vi "RPC Driver Library Path.vi"(8 "Driver ID (\"\")":string, 9 "Driver Type (\"\")":string, 10 "Base Path (empty)":path, 11 "App Ref (null: local)":refnum<vi>) -> (0 "Driver Config Name":string, 1 "Driver Component Name":string, 2 "Driver Library Path":path, 3 "dup App Ref":refnum<vi>)   [LabVIEW 2011]
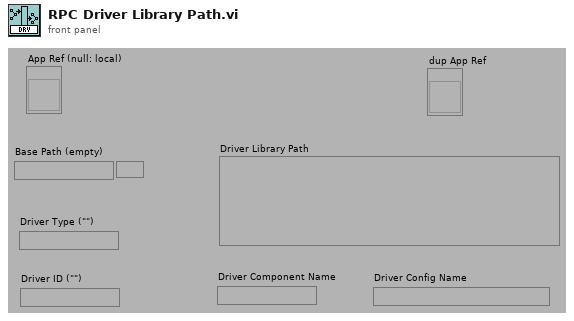
[diagram p1: front panel]
types:
  T1 = enum32{"invalid app kind", "Development System", "Run Time System", "Student Edition", "Embedded LabVIEW", "Evaluation", "Custom"}
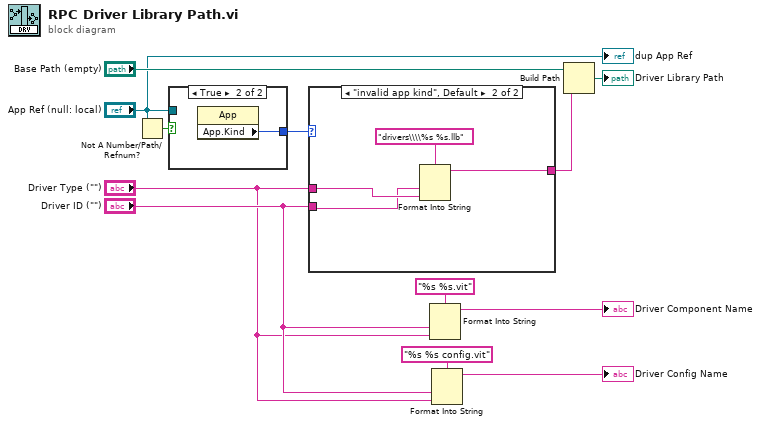
[diagram p0: block diagram]
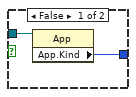
[diagram p2: hidden frame]
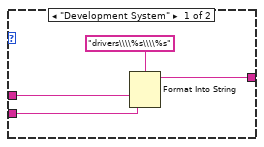
[diagram p3: hidden frame]
diagram:
  n1 = Not A Number/Path/Refnum?(number/path/refnum="App Ref (null: local)") -> (NaN/Path/Refnum?=w1:bool)
  n2 = case shown="True" w1 {
    tunnel: [w14 w15] -> w10
    tunnel: "App Ref (null: local)" -> [w13 _]
    frame False {
      n3 = property class="App"(reference=w13) -> ("App.Kind"=w14:T1)  [unwired: 1 in, 2 out]
    }
    frame True {
      n4 = property class="App"() -> ("App.Kind"=w15:T1)  [unwired: 2 in, 2 out]
    }
  }
  n5 = case shown="\"invalid app kind\", Default" w10 {
    tunnel: [w18 w22] -> w12
    tunnel: "Driver ID (\"\")" -> [w17 w20]
    tunnel: "Driver Type (\"\")" -> [w16 w21]
    frame "Development System" {
      n6 = Format Into String(format string="drivers\\\\%s\\\\%s", w16, w17) -> (resulting string=w18:string)  [unwired: 2 in, 1 out]
    }
    frame "invalid app kind", Default {
      n7 = Format Into String(format string="drivers\\\\%s %s.llb", w20, w21) -> (resulting string=w22:string)  [unwired: 2 in, 1 out]
    }
  }
  n8 = Format Into String(format string="%s %s.vit", "Driver ID (\"\")", "Driver Type (\"\")") -> (resulting string=→"Driver Component Name":string)  [unwired: 2 in, 1 out]
  n9 = Format Into String(format string="%s %s config.vit", "Driver ID (\"\")", "Driver Type (\"\")") -> (resulting string=→"Driver Config Name":string)  [unwired: 2 in, 1 out]
  n10 = Build Path(base path="Base Path (empty)", name or relative path=w12) -> (appended path=→"Driver Library Path":path)
  "dup App Ref" <- "App Ref (null: local)"
